vi "Main VI.vi"(7 "Enum":T2, 8 "error in (no error)":errorcluster) -> (0 "error out":errorcluster, 3 "Queues":T1)   [LabVIEW 2023, in "Internal Communication.lvlib"]
uses:
  Internal Communication.lvlib
  Controls/State FGV.ctl
  Controls/Queues Control.ctl
  Downloads/ATM (100528-01)/ATM (100528-01)/Omi-One Solution/Inner Process Communication/Message.ctl
  Downloads/ATM (100528-01)/ATM (100528-01)/Omi-One Solution/Inner Process Communication/Innes Process Communication.lvlib
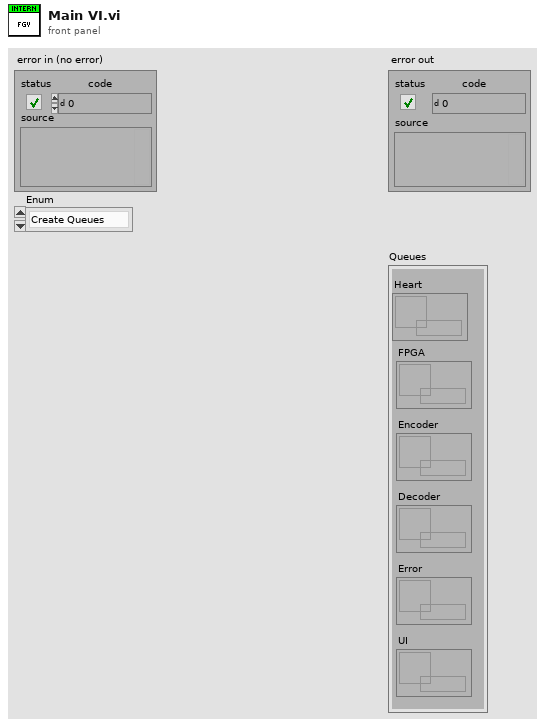
[diagram p1: front panel]
types:
  T1 = typedef "Internal Communication.lvlib/Queues Control.ctl" = cluster{"Heart":refnum<queue>, "FPGA":refnum<queue>, "Encoder":refnum<queue>, "Decoder":refnum<queue>, "Error":refnum<queue>, "UI":refnum<queue>}
  T2 = typedef "Internal Communication.lvlib/State FGV.ctl" = enum16{"Create Queues", "Get Queues", "Destroy Queues"}
  T3 = typedef "Innes Process Communication.lvlib/Message.ctl" = cluster{"Command":string, "Data":variant}
  T4 = cluster{"Display Console Queue":refnum<queue>, "ATM Controller Queue":refnum<queue>, "User Console Queue":refnum<queue>, "Sensor Interface Queue":refnum<queue>, "Configuration Database Queue":refnum<queue>, "Error Handling Queue":refnum<queue>}
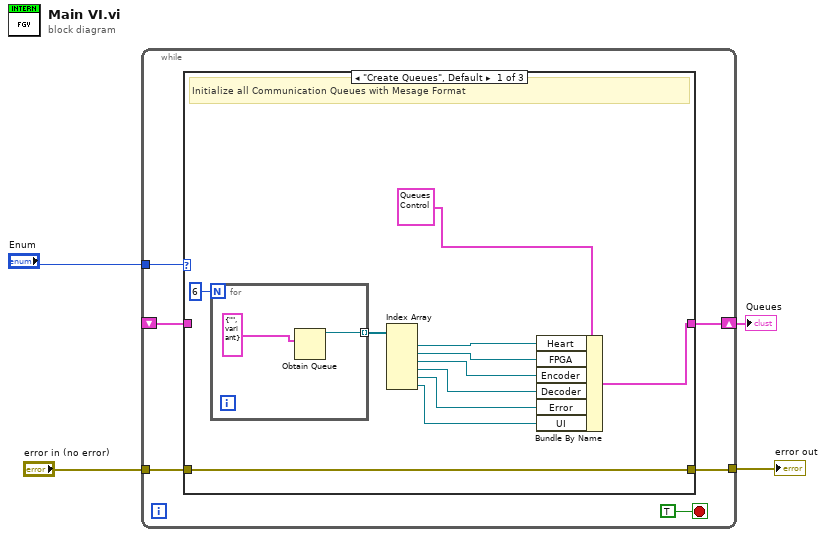
[diagram p0: block diagram]
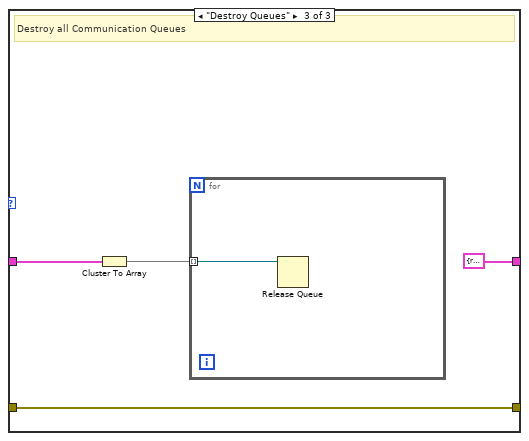
[diagram p3: hidden frame]
diagram:
  n1 = while {
    shift-right: [w10] -> w1
    shift-left: _ -> [w7]
    tunnel: "Enum" -> [w8]
    tunnel: [w6] -> w3
    tunnel: "error in (no error)" -> [w5]
    stop <- TRUE stop-if-true
    n2 = case shown="\"Create Queues\", Default" w8 {
      tunnel: [w20 w25 T4 {"Display Console Queue"=refnum, "ATM Controller Queue"=refnum, "User Console Queue"=refnum, "Sensor Interface Queue"=refnum, "Configuration Database Queue"=refnum, "Error Handling Queue"=refnum} ("Inner Process Queues Cluester")] -> w10
      tunnel: w7 -> [_ w25 w29]
      tunnel: [w18 w24 w26] -> w6
      tunnel: w5 -> [w18 w24 w26]
      frame "Create Queues", Default {
        # "Initialize all Communication Queues with Mesage Format"
        n3 = for {
          N: 6 -> [_]
          tunnel: [w23] -> w21 mode=indexing
          n4 = Obtain Queue(element data type=T3 {"Command"="", "Data"=variant} ("Message")) -> (queue out=w23:refnum<queue>)  [unwired: 4 in, 2 out]
        }
        n5 = Index Array(array=w21) -> (element #1=w17:refnum<queue>, element #2=w16:refnum<queue>, element #3=w15:refnum<queue>, element #4=w14:refnum<queue>, element #5=w13:refnum<queue>, element #6=w12:refnum<queue>)  [unwired: 6 in]
        n6 = Bundle By Name(cluster=T1 {"Heart"=refnum, "FPGA"=refnum, "Encoder"=refnum, "Decoder"=refnum, "Error"=refnum, "UI"=refnum} ("Queues"), "Heart"=w17, "FPGA"=w16, "Encoder"=w15, "Decoder"=w14, "Error"=w13, "UI"=w12) -> (w20:T1)
      }
      frame "Get Queues" {
        # "Get all Communication Queues"
      }
      frame "Destroy Queues" {
        # "Destroy all Communication Queues"
        n7 = Cluster To Array(cluster=w29) -> (array=w28:refnum<queue>[])
        n8 = for {
          tunnel: w28 -> [w30] mode=indexing
          n9 = Release Queue(queue=w30) -> ()  [unwired: 2 in, 3 out]
        }
      }
    }
  }
  "error out" <- w3
  "Queues" <- w1
